vi "Read.vi"(8 "error in (no error)":errorcluster, 11 "Transition Command Config in":refnum<class "Transition Command Config.lvclass">) -> (0 "error out":errorcluster, 2 "Target":string, 3 "Transition Command Config out":refnum<class "Transition Command Config.lvclass">)   [LabVIEW 2020, in "VolatusSeqConfig.lvlib" / "Transition Command Config.lvclass"]
uses:
  Transition Command Config.lvclass
  Transition Command Config.lvclass/Transition Command Config.ctl
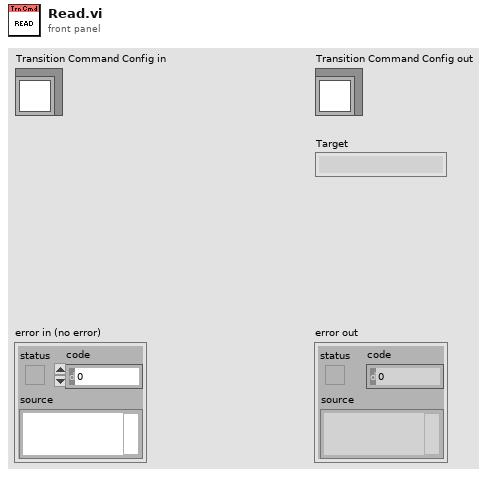
[diagram p1: front panel]
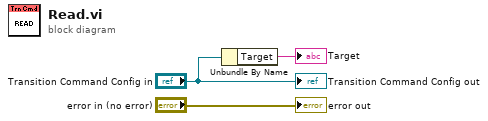
[diagram p0: block diagram]
diagram:
  n1 = Unbundle By Name("Transition Command Config in") -> ("Target"=→"Target":string)
  "error out" <- "error in (no error)"
  "Transition Command Config out" <- "Transition Command Config in"
